vi "tempCreate.vi"(11 "Dev Actor Panel in":refnum<class "Dev Panel.lvclass">) -> (0 "error out":errorcluster, 3 "Dev Actor Panel out":refnum<class "Dev Panel.lvclass">)   [LabVIEW 2021, in "Dev Panel.lvclass"]
uses:
  Dev Panel.lvclass
  Dev Panel.lvclass/Dev Panel.ctl
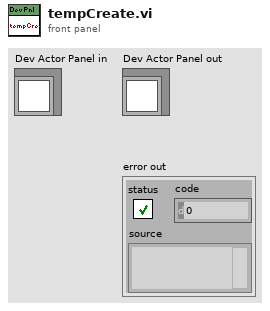
[diagram p1: front panel]
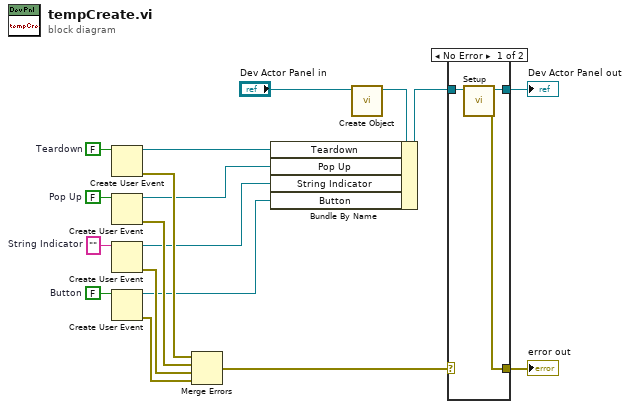
[diagram p0: block diagram]
diagram:
  w13 = FALSE  # Pop Up
  w14 = FALSE  # Button
  w15 = ""  # String Indicator
  w18 = FALSE  # Teardown
  n1 = Create User Event(user event datatype=w18) -> (user event=w17:refnum<user-event>, error out=w16:errorcluster)  [unwired: 1 in]
  n2 = Create User Event(user event datatype=w13) -> (user event=w9:refnum<user-event>, error out=w12:errorcluster)  [unwired: 1 in]
  n3 = Create User Event(user event datatype=w15) -> (user event=w8:refnum<user-event>, error out=w10:errorcluster)  [unwired: 1 in]
  n4 = Create User Event(user event datatype=w14) -> (user event=w7:refnum<user-event>, error out=w11:errorcluster)  [unwired: 1 in]
  n5 = Merge Errors(w16, w12, w10, w11) -> (w4:errorcluster)
  n6 = call "Create Object.vi"("Dev Panel in"="Dev Actor Panel in") -> ("Dev Panel out"=w1:refnum<class "Dev Panel.lvclass">)  [unwired: 10 in]
  n7 = Bundle By Name(cluster=w1, "Teardown"=w17, "Pop Up"=w9, "String Indicator"=w8, "Button"=w7) -> (w6:refnum<class "Dev Panel.lvclass">)
  n8 = case shown="No Error" w4 {
    selector: w4 -> [_ w23]
    tunnel: w6 -> [w21 w22]
    tunnel: [w20 w22] -> w5
    tunnel: [w19 w23] -> w3
    frame No Error {
      n9 = call "Setup.vi"("Dev Panel in"=w21) -> ("error out"=w19:errorcluster, "Dev Panel out"=w20:refnum<class "Dev Panel.lvclass">)  [unwired: 9 in]
    }
    frame Error {
    }
  }
  "error out" <- w3
  "Dev Actor Panel out" <- w5
